vi "Test Serialize Timestamps.vi"(8 "error in (no error)":errorcluster) -> (0 "error out":errorcluster)   [LabVIEW 2013]
uses:
  src/Serializer/JSON Serializer/JSON Serializer.lvclass
  <vilib>/addons/_JKI Toolkits/Caraya/classes/Test/Test.lvclass
  <vilib>/addons/_JKI Toolkits/Caraya/classes/Assert/Assert.lvclass
  src/Deserializer/JSON Deserializer/JSON Deserializer.lvclass
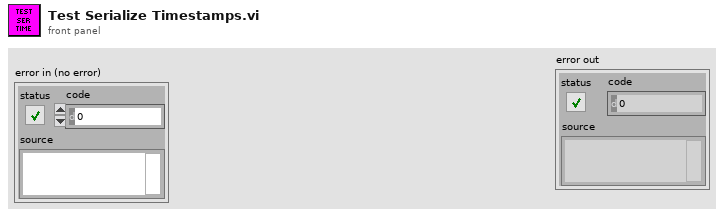
[diagram p1: front panel]
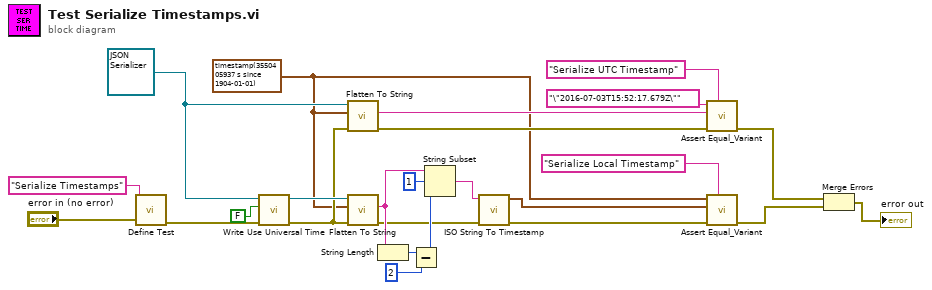
[diagram p0: block diagram]
diagram:
  w8 = timestamp(3550405937.679 s since 1904-01-01)
  w15 = refnum<class "JSON Serializer.lvclass"> refnum ("JKI JSON Serialization.lvlib:JSON Serializer.lvclass")
  n1 = call <vilib>:"Define Test.vi"("error in (no error)"="error in (no error)", "Label (VI Title)"="Serialize Timestamps") -> ("error out"=w13:errorcluster)  [unwired: 9 in]
  n2 = call-dynamic "Write Use Universal Time.vi"("error in (no error)"=w13, "Universal Time"=FALSE, "JSON Serializer in"=w15) -> ("error out"=w12:errorcluster, "JSON Serializer out"=w14:refnum<class "JSON Serializer.lvclass">)  [unwired: 7 in]
  n3 = call-dynamic "Flatten To String.vi"("error in (no error)"=w12, "Variant"=w8, "JSON Serializer in"=w15) -> ("error out"=w23:errorcluster, "String"=w22:string)  [unwired: 6 in, 1 out]
  n4 = call-dynamic "Flatten To String.vi"("error in (no error)"=w12, "Variant"=w8, "JSON Serializer in"=w14) -> ("error out"=w1:errorcluster, "String"=w7:string)  [unwired: 6 in, 1 out]
  n5 = String Length(string=w7) -> (length=w6:i32)
  n6 = Subtract(x=w6, y=2) -> (x-y=w4:i32)
  n7 = String Subset(string=w7, offset (0)=1, length (rest)=w4) -> (substring=w2:string)
  n8 = call "ISO String To Timestamp.vi"("error in (no error)"=w1, "ISO Timestamp String"=w2) -> ("error out"=w10:errorcluster, "Time Stamp"=w9:timestamp)  [unwired: 8 in]
  n9 = call <vilib>:"Assert Equal_Variant.vi"("Label"="Serialize UTC Timestamp", "error in (no error)"=w23, "Y"=w22, "X"="\"2016-07-03T15:52:17.679Z\"") -> ("error out"=w17:errorcluster)  [unwired: 7 in]
  n10 = call <vilib>:"Assert Equal_Variant.vi"("Label"="Serialize Local Timestamp", "error in (no error)"=w10, "Y"=w9, "X"=w8) -> ("error out"=w18:errorcluster)  [unwired: 7 in]
  n11 = Merge Errors(w17, w18) -> (→"error out":errorcluster)
